vi "Image Type key.vi"() -> (3 "String":string)   [LabVIEW 2020, in "SimpleDependencyInspector.lvlib"]
uses:
  SimpleDependencyInspector.lvlib
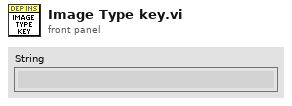
[diagram p1: front panel]
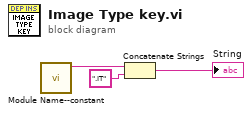
[diagram p0: block diagram]
diagram:
  n1 = call "Module Name--constant.vi"() -> ("Module Name"=w1:string)  [unwired: 11 in]
  n2 = Concatenate Strings(w1, ".IT" ("string")) -> (→"String":string)
